vi "Covert_adc_to_real_value.vi"(11 "ADC":i32) -> (1 "Resistencia":dbl, 2 "Corriente":dbl, 3 "Voltaje":dbl)   [LabVIEW 2019, in "Analisis.lvlib"]
doc: "In this SubVI the adc value is transformed to real value, in this case, depending the adc value is te value of the voltage and resistance"
uses:
  Analisis.lvlib
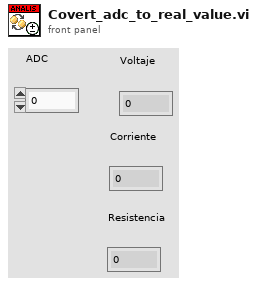
[diagram p1: front panel]
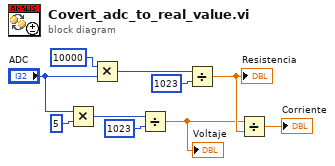
[diagram p0: block diagram]
diagram:
  n1 = Multiply(x="ADC", y=5) -> (x*y=w2:i32)
  n2 = Multiply(x=10000, y="ADC") -> (x*y=w6:i32)
  n3 = Divide(x=w2, y=1023) -> (x/y=w8:dbl)
  "Voltaje" <- w8
  n4 = Divide(x=w6, y=1023) -> (x/y=w9:dbl)
  "Resistencia" <- w9
  n5 = Divide(x=w8, y=w9) -> (x/y=→"Corriente":dbl)
